vi "RotatationTest.vi"() -> ()   [LabVIEW 2022 SP3]
uses:
  <vilib>/Motion/FlexMotion/FunctionsVIs/StartStopMotion.llb/Start Motion (8 axes).flx
  <vilib>/Motion/FlexMotion/FunctionsVIs/Trajectory.llb/Load Acceleration/Deceleration.flx
  <vilib>/Motion/FlexMotion/FunctionsVIs/OnboardProgramming.llb/Wait on Condition (8 axes).flx
  <vilib>/Motion/FlexMotion/CustomControls/CustomControls.llb/Program.flx
  <vilib>/Motion/FlexMotion/CustomControls/CustomControls.llb/Axis To Read.flx
panel:
  out "error out":errorcluster
  out "Store Loop":i32
  in  "Total steps":i32=80000000
  out "Start Position":i32
  in  "error in (no error)":errorcluster
  in  "Axis":T1=4 items=["Axis 1"=1, "Axis 2"=2, "Axis 3"=3, "Axis 4"=4, "Axis 5"=5, "Axis 6"=6, "Axis 7"=7, "Axis 8"=8]
  in  "Program (1)":T2=8 format="%.0x"
  in  "Board ID":T3=1 min=1 max=32 step=1
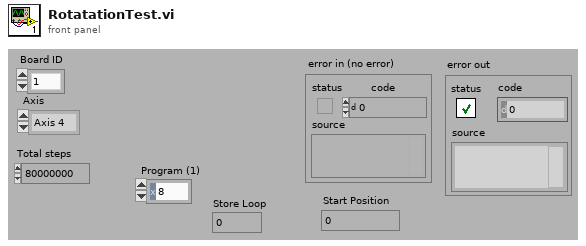
[diagram p1: front panel]
types:
  T1 = typedef "Axis To Read.flx" = u16
  T2 = typedef "Program.flx" = u8
  T3 = typedef "Board Id" = u8
  T4 = enum16{"No Change", "Reset on Breakpoint", "Set on Breakpoint", "Toggle on Breakpoint", "Create Pulse on Breakpoint"}
  T5 = enum16{"Absolute Breakpoint", "Relative Breakpoint", "Modulo Breakpoint", "Periodic Breakpoint"}
  T6 = typedef "Bd Id Out" = u8
  T7 = typedef "Resource Out (Enum).flx" = u16
  T8 = cluster{"0":bool, "1":bool, "2":bool, "3":bool, "4":bool, "5":bool, "6":bool, "7":bool, "8":bool}
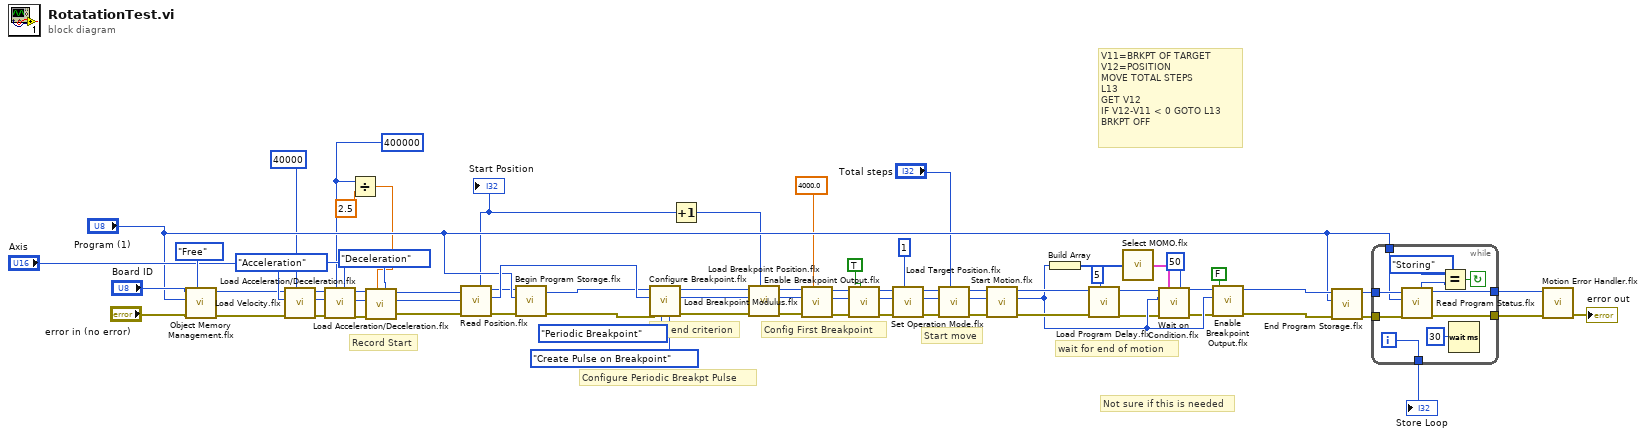
[diagram p0: block diagram]
diagram:
  w20 = 400000 ("motor accel")
  # "wait for end of motion"
  # "Not sure if this is needed"
  # "Configure Periodic Breakpt Pulse"
  # "Set end criterion"
  # "V11=BRKPT OF TARGET\nV12=POSITION\nMOVE TOTAL STEPS\nL13\nGET V12\nIF V12-V11 < 0 GOTO L13\nBRKPT OFF"
  # "Record Start"
  # "Config First Breakpoint"
  # "Start move"
  n1 = call <vilib>:"Object Memory Management.flx"("Operation"=enum16{"Save", "Delete", "Free"}."Free" ("Operation (Free)"), "error in (no error)"="error in (no error)", "Object (1)"="Program (1)", "Board ID"="Board ID") -> ("error out"=w30:errorcluster, "Bd ID Out"=w31:T6)  [unwired: 4 out]
  n2 = call <vilib>:"Load Velocity.flx"("Velocity (10000)"=40000 ("motor velocity"), "error in (no error)"=w30, "Axis or Vector Space"="Axis", "Board ID"=w31) -> ("error out"=w62:errorcluster, "Resource Output"=w60:T7, "Bd ID Out"=w61:T6)  [unwired: 3 out]
  n3 = call "Load Acceleration/Deceleration.flx"("Acceleration Type (Both)"=enum16{"Both", "Acceleration", "Deceleration"}."Acceleration", "Acceleration (100000)"=w20, "error in (no error)"=w62, "Axis or Vector Space"=w60, "Board ID"=w61) -> ("error out"=w25:errorcluster, "Resource Output"=w24:T7, "Bd ID Out"=w28:T6)  [unwired: 2 out]
  n4 = Divide(x=w20, y=2.5) -> (x/y=w19:dbl)
  n5 = call "Load Acceleration/Deceleration.flx"("Acceleration Type (Both)"=enum16{"Both", "Acceleration", "Deceleration"}."Deceleration", "Acceleration (100000)"=w19, "error in (no error)"=w25, "Axis or Vector Space"=w24, "Board ID"=w28) -> ("error out"=w26:errorcluster, "Resource Output"=w23:T7, "Bd ID Out"=w27:T6)  [unwired: 2 out]
  n6 = call <vilib>:"Read Position.flx"("error in (no error)"=w26, "Axis"=w23, "Board ID"=w27) -> ("error out"=w32:errorcluster, "Resource Output"=w41:T7, "Bd ID Out"=w33:T6, "Position"=w7:i32)  [unwired: 3 out]
  "Start Position" <- w7
  n7 = call <vilib>:"Begin Program Storage.flx"("error in (no error)"=w32, "Program (1)"="Program (1)", "Board ID"=w33) -> ("error out"=w3:errorcluster, "Bd ID Out"=w4:T6)  [unwired: 4 out]
  n8 = call <vilib>:"Configure Breakpoint.flx"("Action (No Change)"=T4."Create Pulse on Breakpoint", "Mode (Absolute)"=T5."Periodic Breakpoint", "error in (no error)"=w3, "Axis or Encoder"=w41, "Board ID"=w4) -> ("error out"=w5:errorcluster, "Resource Output"=w51:T7, "Bd ID Out"=w6:T6)  [unwired: 1 in, 3 out]
  n9 = Increment(x=w7) -> (x+1=w1:i32)
  n10 = call <vilib>:"Load Breakpoint Position.flx"("Breakpoint Position (0)"=w1, "error in (no error)"=w5, "Axis or Encoder"=w51, "Board ID"=w6) -> ("error out"=w56:errorcluster, "Resource Output"=w55:T7, "Bd ID Out"=w57:T6)  [unwired: 3 out]
  n11 = call <vilib>:"Load Breakpoint Modulus.flx"("Breakpoint Modulus (0)"=sgl 4000.0 ("Distance between\nscan lines (mm)"), "error in (no error)"=w56, "Axis or Encoder"=w55, "Board ID"=w57) -> ("error out"=w45:errorcluster, "Resource Output"=w46:T7, "Bd ID Out"=w47:T6)  [unwired: 3 out]
  n12 = call <vilib>:"Enable Breakpoint Output.flx"("Enable Breakpoint"=TRUE, "error in (no error)"=w45, "Axis or Encoder"=w46, "Board ID"=w47) -> ("error out"=w44:errorcluster, "Resource Output"=w42:T7, "Bd ID Out"=w43:T6)  [unwired: 3 out]
  n13 = call <vilib>:"Set Operation Mode.flx"("Position Mode (Absolute)"=1, "error in (no error)"=w44, "Axis or Vector Space"=w42, "Board ID"=w43) -> ("error out"=w70:errorcluster, "Resource Output"=w67:T7, "Bd ID Out"=w71:T6)  [unwired: 2 out]
  n14 = call <vilib>:"Load Target Position.flx"("Target Position (0)"="Total steps", "error in (no error)"=w70, "Axis"=w67, "Board ID"=w71) -> ("error out"=w72:errorcluster, "Resource Output"=w73:T7, "Bd ID Out"=w68:T6)  [unwired: 3 out]
  n15 = call-poly <vilib>:"Start Motion.flx"("error in (no error)"=w72, "Axis or Vector Space"=w73, "Board ID"=w68) -> ("error out"=w53:errorcluster, "Resource Output"=w37:T7, "Bd ID Out"=w54:T6)  [unwired: 1 in, 2 out]
  n16 = Build Array(w37) -> (w16:T7[])
  n17 = call <vilib>:"Load Program Delay.flx"("Delay Value (1 ms)"=5, "error in (no error)"=w53, "Board ID"=w54) -> ("error out"=w11:errorcluster, "Bd ID Out"=w12:T6)  [unwired: 4 out]
  n18 = call <vilib>:"Select MOMO.flx"("Resource"=w16) -> ("Must On/Off"=w17:T8)
  n19 = call-poly <vilib>:"Wait on Condition.flx"("Board ID"=w12, "Must On (False)"=w17, "Timeout (1)"=u16 50, "Resource (0)"=w37, "error in (no error)"=w11) -> ("Bd ID Out"=w14:T6, "error out"=w13:errorcluster)  [unwired: 4 in, 5 out]
  n20 = call <vilib>:"Enable Breakpoint Output.flx"("Enable Breakpoint"=FALSE, "error in (no error)"=w13, "Axis or Encoder"=w37, "Board ID"=w14) -> ("error out"=w52:errorcluster, "Bd ID Out"=w35:T6)  [unwired: 4 out]
  n21 = call <vilib>:"End Program Storage.flx"("error in (no error)"=w52, "Program (1)"="Program (1)", "Board ID"=w35) -> ("error out"=w65:errorcluster, "Bd ID Out"=w66:T6)  [unwired: 4 out]
  n22 = while {
    tunnel: w66 -> [w83]
    tunnel: w65 -> [w82]
    tunnel: [w81] -> w40
    tunnel: [w80] -> w39
    tunnel: "Program (1)" -> [w79]
    tunnel: [w75] -> w64
    i -> [w75]
    stop <- w76 continue-if-true
    n23 = call <vilib>:"Read Program Status.flx"("error in (no error)"=w82, "Program (1)"=w79, "Board Id"=w83) -> ("error out"=w80:errorcluster, "Bd Id Out"=w81:T6, "Program Status"=w77:enum16{"Done", "Playing", "Paused", "Storing"})  [unwired: 4 out]
    n24 = Equal?(x=enum16{"Done", "Playing", "Paused", "Storing"}."Storing" ("Program Status"), y=w77) -> (x = y?=w76:bool)
    n25 = Wait (ms)(milliseconds to wait=30) -> ()  [unwired: 1 out]
  }
  "Store Loop" <- w64
  n26 = call <vilib>:"Motion Error Handler.flx"("Board ID"=w40, "error in (no error)"=w39) -> ("error out"=→"error out":errorcluster)  [unwired: 4 in, 9 out]
